vi "Actuator Force Boundary DAO.vi"(7 "refnum in":T1, 8 "error in (no error)":errorcluster, 10 "Limit Boundary Parameters In":T2, 11 "Actions":T3) -> (0 "error out":errorcluster, 2 "Limit Boundary Parameters Out":T2, 4 "refnum out":T1)   [LabVIEW 2013]
uses:
  Metadata/Persistant DAO Actions.ctl
  Limit Boundary Parameters.ctl
  <vilib>/Utility/config.llb/Config Data RefNum.ctl
  <vilib>/Utility/config.llb/NI_LVConfig.lvlib
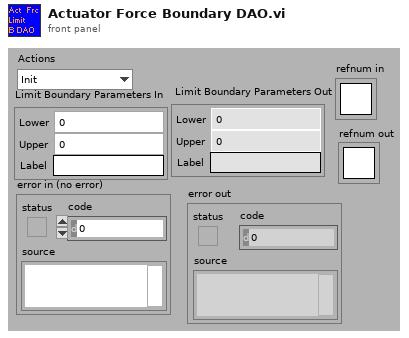
[diagram p1: front panel]
types:
  T1 = typedef "NI_LVConfig.lvlib/Config Data RefNum.ctl" = refnum<k1>
  T2 = typedef "Limit Boundary Parameters.ctl" = cluster{"Lower":dbl, "Upper":dbl, "Label":string}
  T3 = typedef "Persistant DAO Actions.ctl" = enum16{"Init", "Get", "Set", "Load", "Save"}
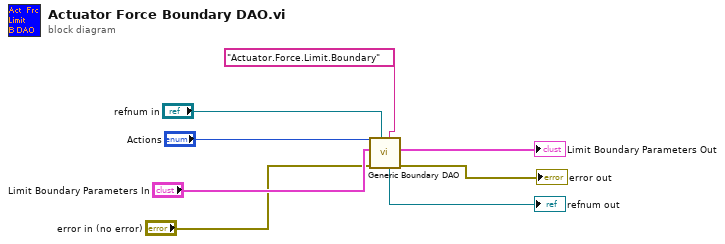
[diagram p0: block diagram]
diagram:
  n1 = call "Generic Boundary DAO.vi"("Section"="Actuator.Force.Limit.Boundary", "refnum in"="refnum in", "error in (no error)"="error in (no error)", "Limit Boundary Parameters In"="Limit Boundary Parameters In", "Persistent DAO Actions"="Actions") -> ("error out"=→"error out":errorcluster, "Limit Boundary Parameters Out"=→"Limit Boundary Parameters Out":T2, "refnum out"=→"refnum out":T1)  [unwired: 4 out]
